vi "Setup Fast F Sweep.vi"(4 "TO, ms":u32=100, 5 "Retry on TO":bool, 7 "Generate F array":bool=TRUE, 8 "error in":errorcluster, 11 "RUS settings in":T1={"NI-DAQ lockin settings"={"Samples per sine wave"=0, "Sine waves per freq step"=0, "Output Representation"=enum."Real/Imaginary", "Low-pass filter"=enum."Butterworth", "Ranges and couplings "=[]}, "Fast swep settings"={"Update rate (Hz)"=250.0, "Start F, Hz"=200000.0, "Stop F"=1700000.0, "Number of points"=30000, "Amplitude"=2.1, "Init&amplitude"=TRUE, "IF"=1000.0, "Time constant"=0.1}, "Pre-sweep delay, s"=0.0, "Lockin mode"=enum."NI-DAQ", "SR Lockin"="GPIB0::10::INSTR", "DAQmx Device"="Dev3", "Clock Multiplier"=64, "Fast Sweep Data Out"={"DO clock task"="", "DO task"="", "Update clock task"="", "DAQ lockin task"="", "Pre-sweep counter task"=""}, "Lockin Range, V"=0.0, "F Array"=[], "Freq. update clock terminal"="", "DO Clock Rate (Hz)"=5000000.0, "ADC clock terminal"="/PFI4", "Pre-sweep counter terminal"="/PFI4", "Samples per read"=10, "DO clock terminal"="", "Pre-sweep points"=0, "F points per write"=0, "Total sweep time, s"=1000.0, "Initial SYNTH phase"=0.0, "Record IF"=FALSE, "Save data settings"={"Save data"=TRUE, "Data Root Path"=path "", "File Prefix"="", "File Format"=enum."ASCII", "Save column names"=TRUE, "File Comments"="<Description of the current file>", "User/Prj"="<User Name/Project Description>"}, "Data file path"=path "", "New data user event"=refnum, "Stop user event"=refnum, "Number of channels"=1, "Auto-phase"=FALSE} {"Lockin Range, V" format="%#_6e"; "Fast swep settings"."IF" format="%#_6p"; "Fast swep settings"."Amplitude" min=0.0 max=2.5; "Fast swep settings"."Number of points" format="%.0p"; "Fast swep settings"."Stop F" format="%#_6p"; "Fast swep settings"."Start F, Hz" format="%#_6p"; "Fast swep settings"."Update rate (Hz)" format="%0.2f"; "NI-DAQ lockin settings"."Ranges and couplings"."Coupling" items=["default"=-1, "RSE"=10083, "NRSE"=10078, "Differential"=10106, "Pseudodifferential"=12529]}) -> (0 "error out":errorcluster, 1 "DO task setup time":u32, 3 "RUS settings out":T1={"NI-DAQ lockin settings"={"Samples per sine wave"=0, "Sine waves per freq step"=0, "Output Representation"=enum."Real/Imaginary", "Low-pass filter"=enum."Butterworth", "Ranges and couplings "=[]}, "Fast swep settings"={"Update rate (Hz)"=250.0, "Start F, Hz"=200000.0, "Stop F"=1700000.0, "Number of points"=30000, "Amplitude"=2.1, "Init&amplitude"=TRUE, "IF"=1000.0, "Time constant"=0.1}, "Pre-sweep delay, s"=0.0, "Lockin mode"=enum."NI-DAQ", "SR Lockin"="GPIB0::10::INSTR", "DAQmx Device"="Dev3", "Clock Multiplier"=64, "Fast Sweep Data Out"={"DO clock task"="", "DO task"="", "Update clock task"="", "DAQ lockin task"="", "Pre-sweep counter task"=""}, "Lockin Range, V"=0.0, "F Array"=[], "Freq. update clock terminal"="", "DO Clock Rate (Hz)"=5000000.0, "ADC clock terminal"="/PFI4", "Pre-sweep counter terminal"="/PFI4", "Samples per read"=10, "DO clock terminal"="", "Pre-sweep points"=0, "F points per write"=0, "Total sweep time, s"=1000.0, "Initial SYNTH phase"=0.0, "Record IF"=FALSE, "Save data settings"={"Save data"=TRUE, "Data Root Path"=path "", "File Prefix"="", "File Format"=enum."ASCII", "Save column names"=TRUE, "File Comments"="<Description of the current file>", "User/Prj"="<User Name/Project Description>"}, "Data file path"=path "", "New data user event"=refnum, "Stop user event"=refnum, "Number of channels"=1, "Auto-phase"=FALSE} {"Lockin Range, V" format="%#_6e"; "Fast swep settings"."IF" format="%#_6p"; "Fast swep settings"."Amplitude" min=0.0 max=2.5; "Fast swep settings"."Number of points" format="%.0p"; "Fast swep settings"."Stop F" format="%#_6p"; "Fast swep settings"."Start F, Hz" format="%#_6p"; "Fast swep settings"."Update rate (Hz)" format="%0.2f"; "NI-DAQ lockin settings"."Ranges and couplings"."Coupling" items=["default"=-1, "RSE"=10083, "NRSE"=10078, "Differential"=10106, "Pseudodifferential"=12529]})   [LabVIEW 2015]
uses:
  Controls/RUS settings.ctl
  Controls/RUS NI-DAQ Lockin Settings.ctl
  Controls/Sweep settings.ctl
  NHMFL_Core/Libraries/File/Controls/Save data settings.ctl
  NHMFL_Core/Libraries/File/Controls/File formats.ctl
panel:
  out "F1 out time":u32
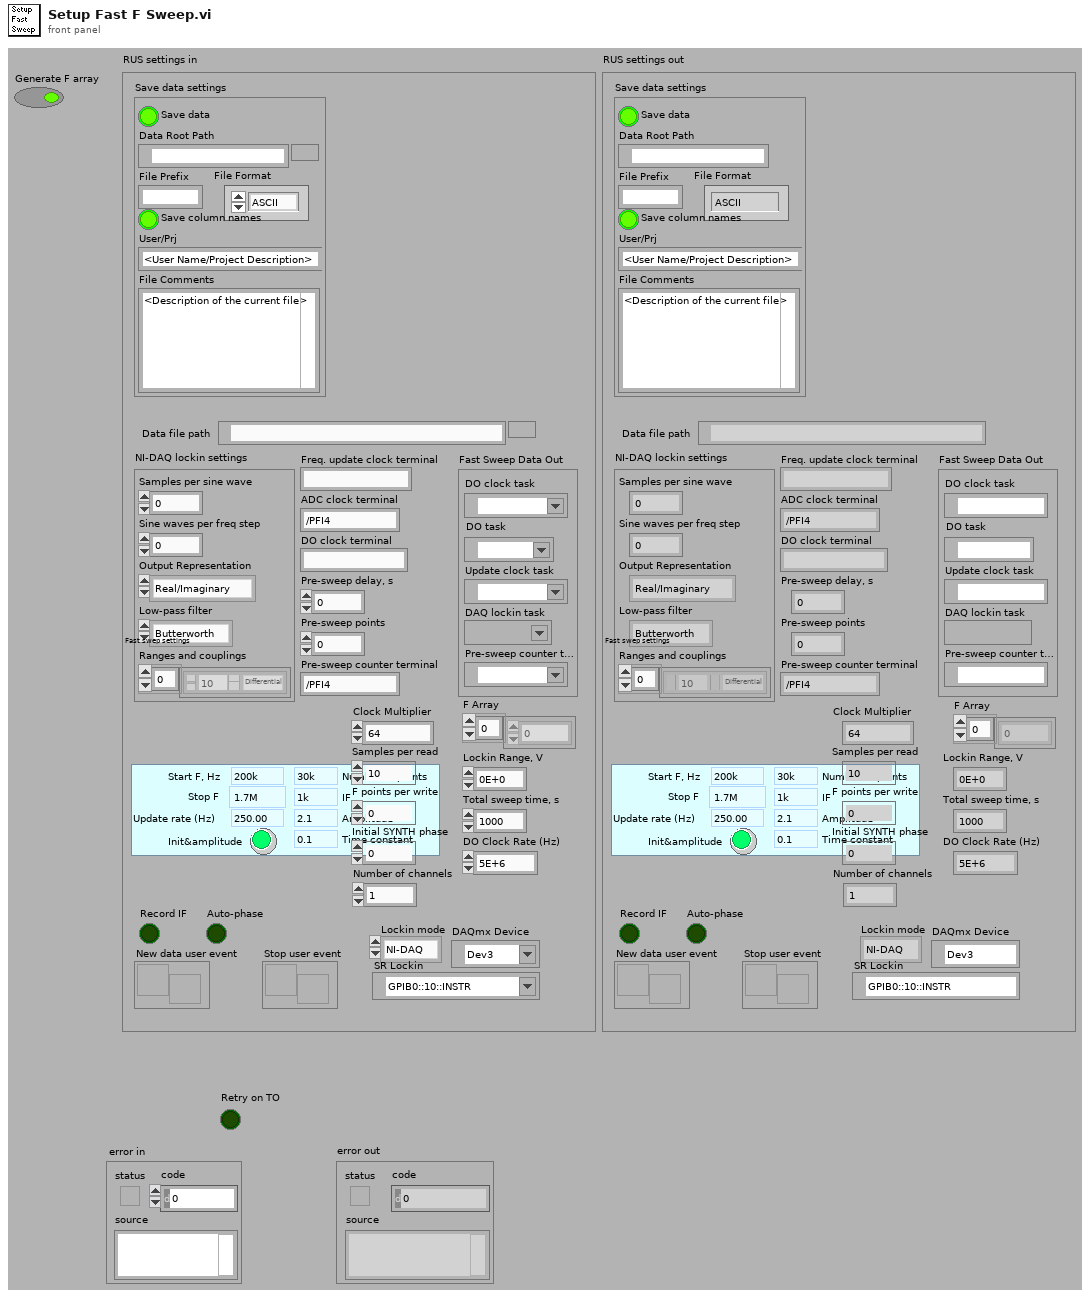
[diagram p1: front panel]
types:
  T1 = typedef "RUS settings.ctl" = cluster{"NI-DAQ lockin settings":T2, "Fast swep settings":T3, "Pre-sweep delay, s":dbl, "Lockin mode":enum16{"SRS", "NI-DAQ"}, "SR Lockin":refnum<visa-resource-name>, "DAQmx Device":tag, "Clock Multiplier":i32, "Fast Sweep Data Out":cluster{"DO clock task":refnum<k21>, "DO task":refnum<k21>, "Update clock task":refnum<k21>, "DAQ lockin task":refnum<k21>, "Pre-sweep counter task":refnum<k21>}, "Lockin Range, V":sgl, "F Array":dbl[], "Freq. update clock terminal":string, "DO Clock Rate (Hz)":dbl, "ADC clock terminal":string, "Pre-sweep counter terminal":string, "Samples per read":i32, "DO clock terminal":string, "Pre-sweep points":i32, "F points per write":i32, "Total sweep time, s":dbl, "Initial SYNTH phase":dbl, "Record IF":bool, "Save data settings":T4, "Data file path":path, "New data user event":refnum<user-event>, "Stop user event":refnum<user-event>, "Number of channels":i32, "Auto-phase":bool}
  T2 = typedef "RUS NI-DAQ Lockin Settings.ctl" = cluster{"Samples per sine wave":i32, "Sine waves per freq step":i32, "Output Representation":enum16{"Real/Imaginary", "Polar"}, "Low-pass filter":enum16{"No filtering", "Butterworth", "Bessel"}, "Ranges and couplings ":cluster{"Range":dbl, "Coupling":i32}[]}
  T3 = typedef "Sweep settings.ctl" = cluster{"Update rate (Hz)":dbl, "Start F, Hz":dbl, "Stop F":dbl, "Number of points":i32, "Amplitude":dbl, "Init&amplitude":bool, "IF":dbl, "Time constant":dbl}
  T4 = typedef "Save data settings.ctl" = cluster{"Save data":bool, "Data Root Path":path, "File Prefix":string, "File Format":T5, "Save column names":bool, "File Comments":string, "User/Prj":string}
  T5 = typedef "File formats.ctl" = enum16{"TDMS", "ASCII", "BINARY"}
  T6 = enum16{"Direct, clock*f1", "Direct, clock*f2", "Heterodyne"}
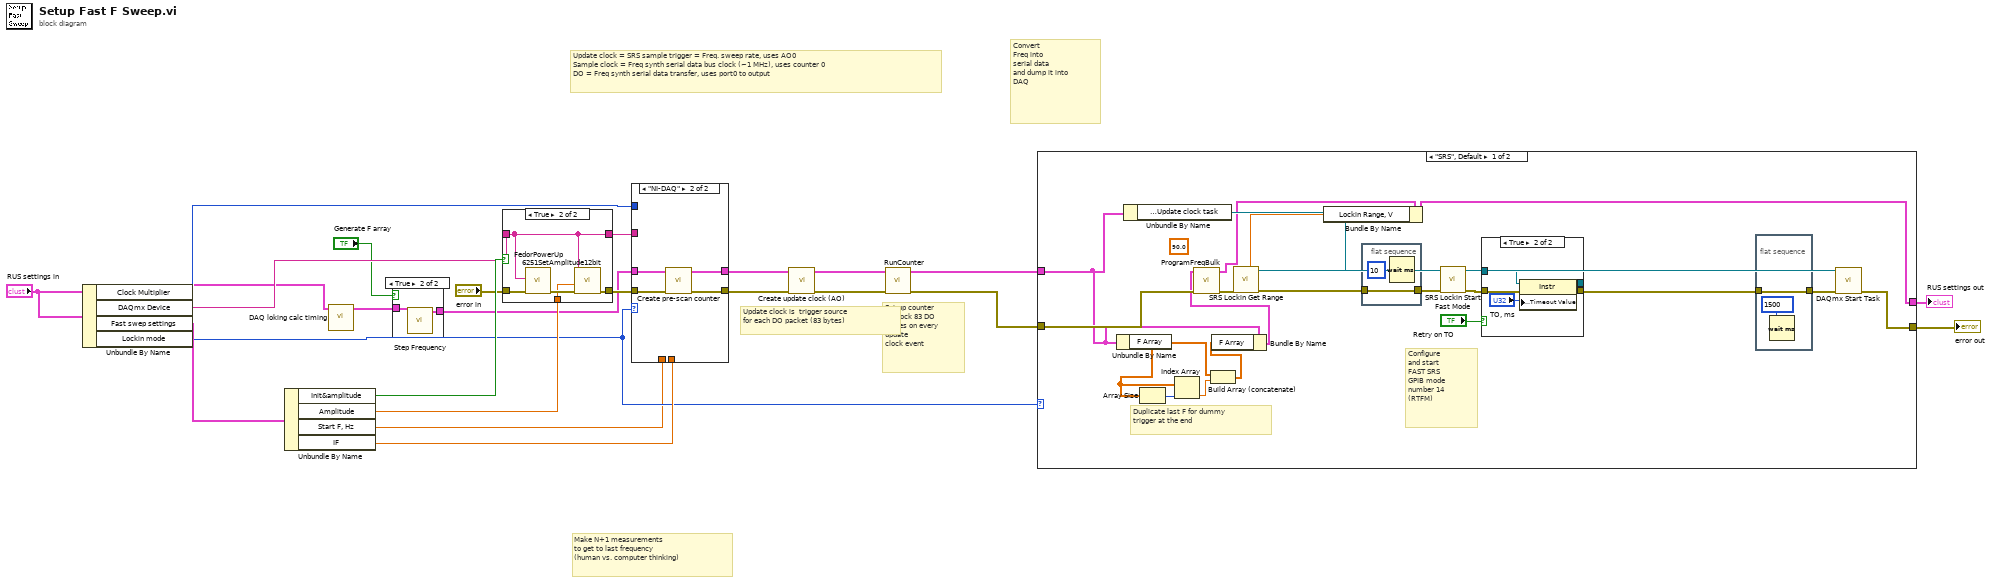
[diagram p0: block diagram]
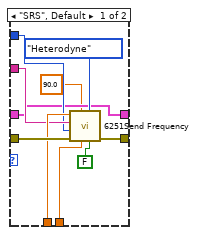
[diagram p3: hidden frame]
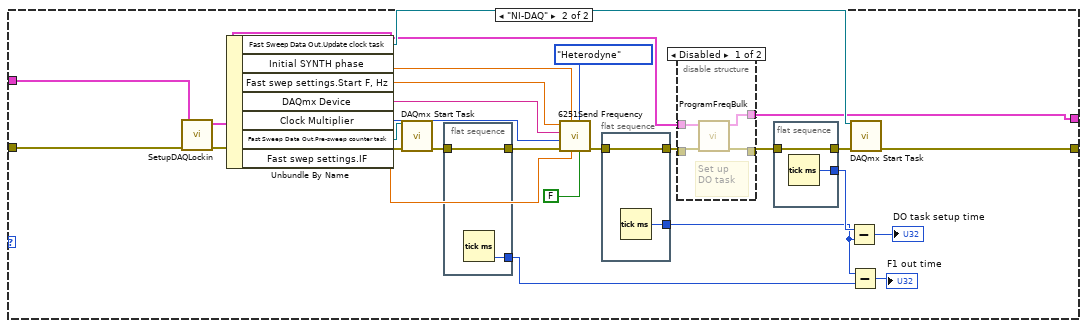
[diagram p5: hidden frame]
diagram:
  # "Make N+1 measurements\nto get to last frequency\n(human vs. computer thinking)"
  # "Set up counter\nto clock 83 DO\ncycles on every\nupdate \nclock event"
  # "Convert \nFreq into \nserial data \nand dump it into \nDAQ"
  # "Update clock is  trigger source\nfor each DO packet (83 bytes)"
  # "Update clock = SRS sample trigger = Freq. sweep rate, uses AO0\nSample clock = Freq synth serial data bus clock (~1 MHz), uses counter 0\nDO = Freq synth serial data transfer, uses port0 to output"
  n1 = Unbundle By Name("RUS settings in") -> ("Clock Multiplier"=w9:i32, "DAQmx Device"=w12:tag, "Fast swep settings"=w14:T3, "Lockin mode"=w13:enum16{"SRS", "NI-DAQ"})
  n2 = Unbundle By Name(w14) -> ("Init&amplitude"=w22:bool, "Amplitude"=w23:dbl, "Start F, Hz"=w7:dbl, "IF"=w17:dbl)
  n3 = call "DAQ loking calc timing.vi"("RUS settings"="RUS settings in") -> ("RUS settings out"=w5:T1)  [unwired: 10 in]
  n4 = case shown="True" "Generate F array" {
    tunnel: w5 -> [w24 w26]
    tunnel: [w24 w25] -> w3
    frame False {
    }
    frame True {
      n5 = call "Step Frequency.vi"("RUS settings"=w26) -> ("RUS settings out"=w25:T1)  [unwired: 3 in, 7 out]
    }
  }
  n6 = case shown="True" w22 {
    tunnel: "error in" -> [w28 w33]
    tunnel: [w28 w31] -> w20
    tunnel: w12 -> [w27 w30]
    tunnel: [w27 w30] -> w18
    tunnel: w23 -> [_ w29]
    frame False {
    }
    frame True {
      n7 = call "FedorPowerUp.vi"("error in (no error)"=w33, "DAQmx Device Name"=w30) -> ("error out"=w32:errorcluster)  [unwired: 9 out]
      n8 = call "6251SetAmplitude12bit.vi"("error in (no error)"=w32, "0 to 2.1 VRMS"=w29, "DAQmx Device Name"=w30) -> ("error out"=w31:errorcluster)  [unwired: 8 out]
    }
  }
  n9 = case shown="\"NI-DAQ\"" w13 {
    tunnel: w20 -> [w43 w47]
    tunnel: [w42 w46] -> w4
    tunnel: w17 -> [w41 _]
    tunnel: w7 -> [w39 _]
    tunnel: w18 -> [w38 _]
    tunnel: w9 -> [w37 _]
    tunnel: w3 -> [w35 w45]
    tunnel: [w35 w44] -> w2
    frame "SRS", Default {
      n10 = call "6251Send Frequency.vi"("Use hardware clock for DO"=FALSE ("6251"), "Mode"=T6."Heterodyne", "IF (Hz)"=w41, "Phase (degrees)"=90.0, "error in (no error)"=w43, "Clock Multiplier"=w37, "DAQmx Device Name"=w38, "f (Hz)"=w39) -> ("error out"=w42:errorcluster)  [unwired: 2 in, 1 out]
    }
    frame "NI-DAQ" {
      n11 = call "Create pre-scan counter.vi"("error in"=w47, "RUS settings"=w45) -> ("error out"=w46:errorcluster, "RUS settings out"=w44:T1)  [unwired: 8 in]
    }
  }
  n12 = call "Create update clock (AO).vi"("error in"=w4, "RUS settings"=w2) -> ("error out"=w19:errorcluster, "RUS settings out"=w11:T1)  [unwired: 3 in, 5 out]
  n13 = call "RunCounter.vi"("error in (no error)"=w19, "RUS settings"=w11) -> ("error out"=w16:errorcluster, "RUS settings out"=w10:T1)  [unwired: 2 in, 6 out]
  n14 = case shown="\"SRS\", Default" w13 {
    tunnel: w16 -> [w55 w105]
    tunnel: [w59 w91] -> w15
    tunnel: w10 -> [w50 w80]
    tunnel: [w57 w86] -> w6
    frame "SRS", Default {
      (unwired) 90.0 ("Phase (degrees)")
      # "Duplicate last F for dummy \ntrigger at the end"
      # "Configure \nand start \nFAST SRS\nGPIB mode\nnumber 14\n(RTFM)"
      n15 = Unbundle By Name(w50) -> ("F Array"=w51:dbl[])
      n16 = Unbundle By Name(w50) -> ("Fast Sweep Data Out.Update clock task"=w58:refnum<k21>)
      n17 = Array Size(array=w51) -> (size(s)=w52:i32)
      n18 = Index Array(array=w51, index=w52) -> (element=w53:dbl)
      n19 = Build Array (concatenate)(w51, w53) -> (w49:dbl[])
      n20 = Bundle By Name(cluster=w50, "F Array"=w49) -> (w48:T1)
      n21 = call "ProgramFreqBulk.vi"("error in (no error)"=w55, "RUS settings"=w48) -> ("error out"=w62:errorcluster, "RUS settings out"=w54:T1)  [unwired: 3 in, 5 out]
      n22 = call "SRS Lockin Get Range.vi"("error in (no error)"=w62) -> ("error out"=w64:errorcluster, "VISA resource name out"=w68:refnum<visa-resource-name>, "Range, V"=w56:sgl)  [unwired: 1 in, 7 out]
      n23 = Bundle By Name(cluster=w54, "Lockin Range, V"=w56) -> (w57:T1)
      n24 = flat-sequence {
        tunnel: w64 -> [w72]
        tunnel: [w72] -> w63
        frame #0 {
          n25 = Wait (ms)(milliseconds to wait=u32 10) -> ()  [unwired: 1 out]
        }
      }
      n26 = call "SRS Lockin Start Fast Mode.vi"("error in (no error)"=w63, "VISA Resource Name"=w68) -> ("error out"=w67:errorcluster, "VISA resource name out"=w65:refnum<visa-resource-name>)  [unwired: 1 in, 7 out]
      n27 = case shown="True" "Retry on TO" {
        tunnel: w67 -> [w74 w79]
        tunnel: [w74 w78] -> w61
        tunnel: w65 -> [w73 w76]
        tunnel: [w73 w75] -> _
        frame False {
        }
        frame True {
          n28 = property class="Instr"(reference=w76, error in=w79, "General Settings:Timeout Value"="TO, ms") -> (reference out=w75:refnum<visa-resource-name>, error out=w78:errorcluster)
        }
      }
      n29 = flat-sequence {
        tunnel: w61 -> [w70]
        tunnel: [w70] -> w60
        frame #0 {
          n30 = Wait (ms)(milliseconds to wait=u32 1500) -> ()  [unwired: 1 out]
        }
      }
      n31 = call <vilib>:"DAQmx Start Task.vi"("task/channels in"=w58, "error in"=w60) -> ("error out"=w59:errorcluster)  [unwired: 13 out]
    }
    frame "NI-DAQ" {
      n32 = call "SetupDAQLockin.vi"("error in (no error)"=w105, "RUS settings"=w80) -> ("error out"=w92:errorcluster, "RUS settings out"=w87:T1)  [unwired: 8 in]
      n33 = Unbundle By Name(w87) -> ("Fast Sweep Data Out.Update clock task"=w90:refnum<k21>, "Initial SYNTH phase"=w81:dbl, "Fast swep settings.Start F, Hz"=w84:dbl, "DAQmx Device"=w89:tag, "Clock Multiplier"=w83:i32, "Fast Sweep Data Out.Pre-sweep counter task"=w93:refnum<k21>, "Fast swep settings.IF"=w85:dbl)
      n34 = call <vilib>:"DAQmx Start Task.vi"("task/channels in"=w93, "error in"=w92) -> ("error out"=w98:errorcluster)  [unwired: 13 out]
      n35 = flat-sequence {
        tunnel: w98 -> [w113]
        tunnel: [w113] -> w97
        tunnel: [w112] -> w95
        frame #0 {
          n36 = Tick Count (ms)() -> (millisecond timer value=w112:u32)
        }
      }
      n37 = call "6251Send Frequency.vi"("Use hardware clock for DO"=FALSE ("6251"), "Mode"=T6."Heterodyne", "IF (Hz)"=w85, "Phase (degrees)"=w81, "error in (no error)"=w97, "Clock Multiplier"=w83, "DAQmx Device Name"=w89, "f (Hz)"=w84) -> ("error out"=w102:errorcluster)  [unwired: 2 in, 1 out]
      n38 = flat-sequence {
        tunnel: w102 -> [w117]
        tunnel: [w117] -> w88
        tunnel: [w116] -> w82
        frame #0 {
          n39 = Tick Count (ms)() -> (millisecond timer value=w116:u32)
        }
      }
      n40 = disable-structure shown="Disabled" {
        disable-tunnel: [w109 w110] -> w101
        disable-tunnel: w88 -> [w108 w110]
        disable-tunnel: w87 -> [w107 w111]
        disable-tunnel: [w106 w111] -> w86
        frame Disabled {
          # "Set up\nDO task"
          n41 = call "ProgramFreqBulk.vi"("error in (no error)"=w108, "RUS settings"=w107) -> ("error out"=w109:errorcluster, "RUS settings out"=w106:T1)  [unwired: 3 in, 5 out]
        }
        frame Enabled {
        }
      }
      n42 = flat-sequence {
        tunnel: w101 -> [w115]
        tunnel: [w115] -> w100
        tunnel: [w114] -> w96
        frame #0 {
          n43 = Tick Count (ms)() -> (millisecond timer value=w114:u32)
        }
      }
      n44 = Subtract(x=w96, y=w82) -> (x-y=→"DO task setup time":u32)
      n45 = Subtract(x=w82, y=w95) -> (x-y=→"F1 out time":u32)
      n46 = call <vilib>:"DAQmx Start Task.vi"("task/channels in"=w90, "error in"=w100) -> ("error out"=w91:errorcluster)  [unwired: 12 in, 1 out]
    }
  }
  "error out" <- w15
  "RUS settings out" <- w6
